vi "TestLoop Manage Queuess.vi"() -> ()   [LabVIEW 2013]
uses:
  My circular buffer info.ctl
panel:
  in  "bytes to write":i32
  in  "cmd":enum16{"toggle buffers", "data event", "stop"}(ring)
  in  "source event":bool
  in  "stop 2":bool
  in  "Np > P?":bool
  in  "Rd buff Exisits?":bool
  out "archive mode":enum16{"direct", "append"}(ring)
  out "bytes to write":i32
  out "archive file":string
  in  "buffer2 path":path
  in  "buffer1 path":path
  in  "archive directory":path
  in  "num blocks  prior":i32
  in  "num blocks after":i32
  in  "bytes/sample":i32
  in  "samples/block/channel":i32
  in  "number of channels":i32
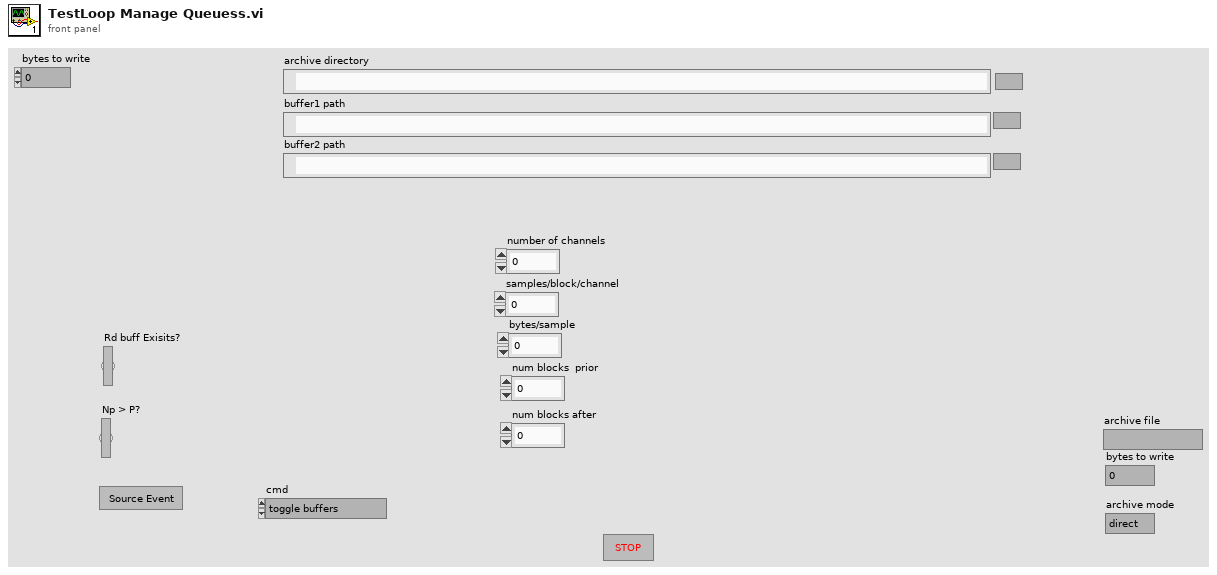
[diagram p1: front panel]
types:
  T1 = typedef "My circular buffer info.ctl" = cluster{"buff ref1":refnum<file>, "buff ref2":refnum<file>, "buffer1 path":path, "buffer2 path":path, "archive directory":path, "xml header":string, "num blocks  prior":i32, "num blocks after":i32, "blocks/event":i32, "samples/block":i32, "bytes/sample":i32, "number of channels":i32, "samples/block/channel":i32, "read buffer ref queue":refnum<queue>, "Event delay queue":refnum<queue>, "command queue":refnum<queue>}
  T2 = cluster{"filename":string, "bytes to write":i32, "archive mode":enum16{"direct", "append"}}
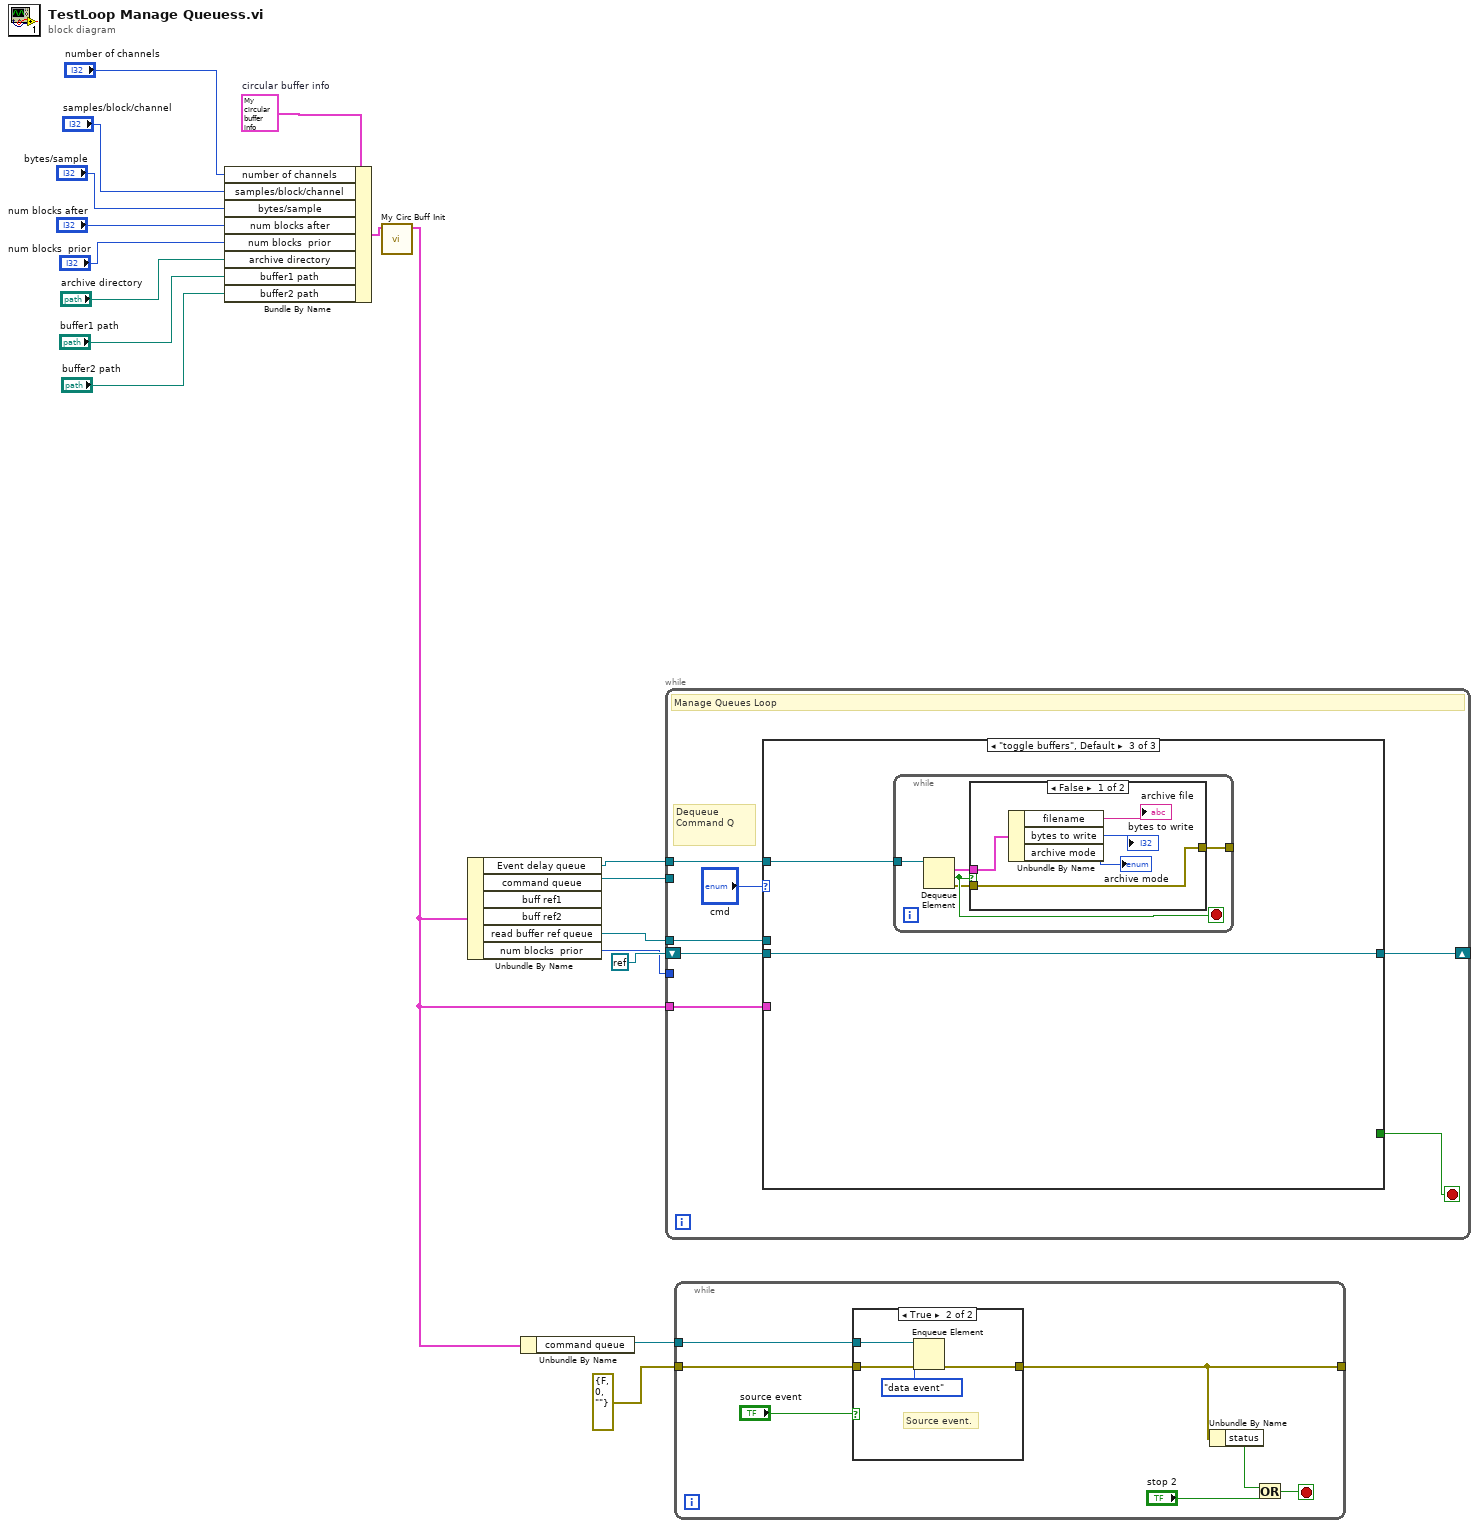
[diagram p0: block diagram]
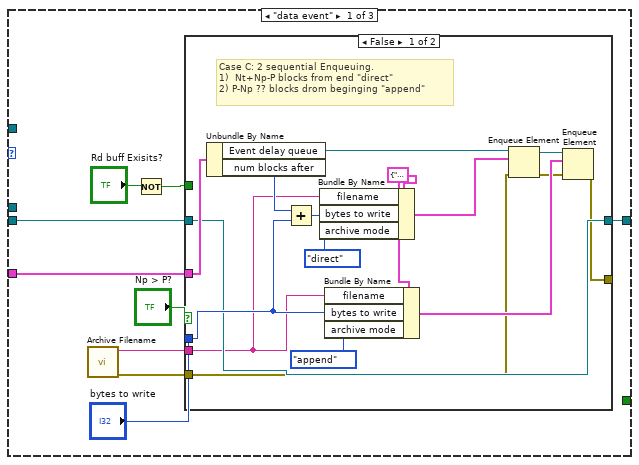
[diagram p3: hidden frame]
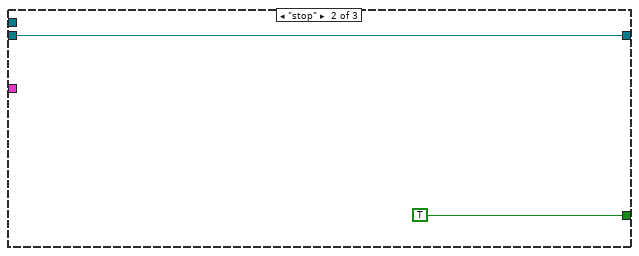
[diagram p6: hidden frame]
diagram:
  w13 = T1 {"buff ref1"=refnum, "buff ref2"=refnum, "buffer1 path"=path "", "buffer2 path"=path "", "archive directory"=path "", "xml header"="", "num blocks  prior"=0, "num blocks after"=0, "blocks/event"=0, "samples/block"=0, "bytes/sample"=0, "number of channels"=0, "samples/block/channel"=0, "read buffer ref queue"=refnum, "Event delay queue"=refnum, "command queue"=refnum}  # circular buffer info
  n1 = Bundle By Name(cluster=w13, "number of channels"="number of channels", "samples/block/channel"="samples/block/channel", "bytes/sample"="bytes/sample", "num blocks after"="num blocks after", "num blocks  prior"="num blocks  prior", "archive directory"="archive directory", "buffer1 path"="buffer1 path", "buffer2 path"="buffer2 path") -> (w9:T1)
  n2 = call "My Circ Buff Init.vi"("circular buffer info"=w9) -> ("circular buffer info out"=w3:T1)  [unwired: 9 in, 1 out]
  n3 = Unbundle By Name(w3) -> ("Event delay queue"=w7:refnum<queue>, "command queue"=w8:refnum<queue>, "read buffer ref queue"=w6:refnum<queue>, "num blocks  prior"=w4:i32)  [unwired: 2 out]
  n4 = Unbundle By Name(w3) -> ("command queue"=w2:refnum<queue>)
  n5 = while {
    tunnel: w8 -> [_]
    shift-right: [w23] -> _
    shift-left: refnum<k0> refnum -> [w25]
    tunnel: w4 -> [_]
    tunnel: w3 -> [w24]
    tunnel: w6 -> [w22]
    tunnel: w7 -> [w21]
    stop <- w19 stop-if-true
    # "Dequeue \nCommand Q"
    # "Manage Queues Loop"
    n6 = case shown="\"toggle buffers\", Default" "cmd" {
      tunnel: w25 -> [w33 w63 w64]
      tunnel: w24 -> [w34 _ _]
      tunnel: [w32 w63 w64] -> w23
      tunnel: w22 -> [_ _ _]
      tunnel: w21 -> [_ _ w65]
      tunnel: [_ TRUE _] -> w19
      frame "data event" {
        n7 = call "Archive Filename.vi"() -> ("error out"=w30:errorcluster, "filename"=w31:string)  [unwired: 10 in]
        n8 = Not(x="Rd buff Exisits?") -> (.not. x?=w27:bool)
        n9 = case shown="False" "Np > P?" {
          tunnel: w27 -> [_ w58]
          tunnel: w34 -> [w40 w57]
          tunnel: "bytes to write" -> [w43 w56]
          tunnel: w33 -> [w39 w55]
          tunnel: [w39 w54] -> w32
          tunnel: w31 -> [w38 w53]
          tunnel: w30 -> [w37 w52]
          tunnel: [w35 w51] -> _
          frame False {
            w42 = T2 {"filename"="", "bytes to write"=0, "archive mode"=enum."direct"} ("Event delay info")
            # "Case C: 2 sequential Enqueuing. \n1)  Nt+Np-P blocks from end \"direct\"\n2) P-Np ?? blocks drom beginging \"append\""
            n10 = Unbundle By Name(w40) -> ("Event delay queue"=w50:refnum<queue>, "num blocks after"=w46:i32)
            n11 = Add(x=w46, y=w43) -> (x+y=w47:i32)
            n12 = Bundle By Name(cluster=w42, "filename"=w38, "bytes to write"=w47, "archive mode"=enum16{"direct", "append"}."direct") -> (w48:T2)
            n13 = Bundle By Name(cluster=w42, "filename"=w38, "bytes to write"=w43, "archive mode"=enum16{"direct", "append"}."append") -> (w41:T2)
            n14 = Enqueue Element(queue=w50, element=w48, error in (no error)=w37) -> (queue out=w45:refnum<queue>, error out=w36:errorcluster)  [unwired: 1 in, 1 out]
            n15 = Enqueue Element(queue=w45, element=w41, error in (no error)=w36) -> (error out=w35:errorcluster)  [unwired: 1 in, 2 out]
          }
          frame True {
            # "Np > Ptr.  Pointer at the begining of Write buffer"
            n16 = case shown="True" w58 {
              tunnel: w57 -> [_ _]
              tunnel: w56 -> [_ _]
              tunnel: w55 -> [_ w61]
              tunnel: [_ w61] -> w54
              tunnel: w53 -> [_ _]
              tunnel: w52 -> [w59 w60]
              tunnel: [w59 w60] -> w51
              frame False {
                # "Case B:  A part of the Nprior data is\nalready in the Read buffer.  \nCopy it to new archive file.\nEnqueue the current Write buffer."
              }
              frame True {
                # "Case A: reference to Read Buffer \ndoes not exisit yet. \nJust enqueue the Read Buff Q (P+Na) blocks."
              }
            }
          }
        }
      }
      frame "stop" {
      }
      frame "toggle buffers", Default {
        n17 = while {
          tunnel: w65 -> [w70]
          tunnel: [w66] -> _
          stop <- w69 stop-if-true
          n18 = Dequeue Element(queue=w70) -> (element=w68:T2, timed out?=w69:bool, error out=w67:errorcluster)  [unwired: 2 in, 1 out]
          n19 = case shown="False" w69 {
            tunnel: w68 -> [w75 _]
            tunnel: w67 -> [w74 w76]
            tunnel: [w74 w76] -> w66
            frame False {
              n20 = Unbundle By Name(w75) -> ("filename"=→"archive file":string, "bytes to write"=→"bytes to write":i32, "archive mode"=→"archive mode":enum16{"direct", "append"})
            }
            frame True {
              # "no event waits"
            }
          }
        }
      }
    }
  }
  n21 = while {
    tunnel: w2 -> [w82]
    tunnel: [w81] -> _
    tunnel: errorcluster {"status"=FALSE, "code"=0, "source"=""} ("error out") -> [w77]
    stop <- w79 stop-if-true
    n22 = case shown="True" "source event" {
      tunnel: w82 -> [_ w88]
      tunnel: [w84 w87] -> w81
      tunnel: w77 -> [w84 w86]
      frame False {
      }
      frame True {
        # "Source event."
        n23 = Enqueue Element(queue=w88, element=enum16{"toggle buffers", "data event", "stop"}."data event", error in (no error)=w86) -> (error out=w87:errorcluster)  [unwired: 1 in, 2 out]
      }
    }
    n24 = Unbundle By Name(w81) -> ("status"=w80:bool)
    n25 = Or(x=w80, y="stop 2") -> (x .or. y?=w79:bool)
  }
